vi "Get LVClass Item Path.vi"(8 "error in (no error)":errorcluster, 11 "LVClassLibrary in":refnum<vi>) -> (0 "error out":errorcluster, 2 "Path":path, 3 "LVClassLibrary out":refnum<vi>)   [LabVIEW 2020, in "gRPC Scripting Tools.lvlib"]
uses:
  gRPC Scripting Tools.lvlib
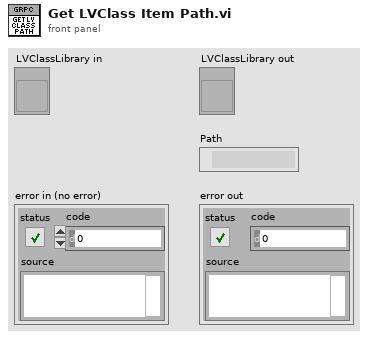
[diagram p1: front panel]
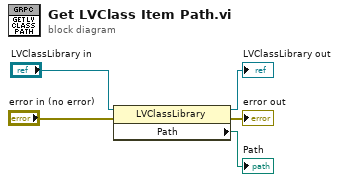
[diagram p0: block diagram]
diagram:
  n1 = property class="LVClassLibrary"(reference="LVClassLibrary in", error in="error in (no error)") -> (reference out=→"LVClassLibrary out":refnum<vi>, error out=→"error out":errorcluster, "Path"=→"Path":path)
